vi "Add Cashier.vi"(7 "Time Scale [ms]":u32=3000, 8 "error in (no error)":errorcluster, 10 "Name":string, 11 "Coffee Shop in":refnum<class "Coffee Shop.lvclass">) -> (0 "error out":errorcluster, 3 "Coffee Shop out":refnum<class "Coffee Shop.lvclass">)   [LabVIEW 2020, in "Coffee Shop.lvclass"]
uses:
  Coffee Shop.lvclass
  C:/Program Files (x86)/National Instruments/LabVIEW 2020/vi.lib/Astemes/Triarc Framework/Process/Process.lvclass
  People/Workers/Cashier/Cashier.lvclass
  C:/git/astemes-triarc-examples/source/Coffee Shop/Processes/People/Person/Person.lvclass
  People/Person/Person.lvclass/Person.ctl
  <vilib>/Astemes/Triarc Framework/Process/Process.lvclass/Process.ctl
  <vilib>/Astemes/Triarc Framework/Process/Private/SubVIs/Handle Debug Data.vi
  <vilib>/Astemes/Triarc Framework/Logging/Log Debug.vi
  <vilib>/AdvancedString/1D String Array to Delimited String.vi
  <vilib>/Utility/High Resolution Relative Seconds.vi
  <vilib>/Astemes/Triarc Framework/Process/Public/Read Name.vi
  <vilib>/Astemes/Triarc Framework/Callback/Callback.lvclass
  Coffee Shop.lvclass/Coffee Shop.ctl
  <vilib>/Astemes/Triarc Framework/Process/Process.lvclass
  C:/git/astemes-triarc-examples/source/Coffee Shop/Processes/People/Workers/Worker/Worker.lvclass
  C:/Program Files (x86)/National Instruments/LabVIEW 2020/vi.lib/Astemes/Triarc Framework/View/View.lvclass
  C:/Program Files (x86)/National Instruments/LabVIEW 2020/vi.lib/Astemes/Triarc Framework/Base/Base.lvclass
  C:/Program Files (x86)/National Instruments/LabVIEW 2020/vi.lib/Astemes/Triarc Framework/Error Handler Interface/Error Handler Interface.lvclass
  C:/Program Files (x86)/National Instruments/LabVIEW 2020/vi.lib/Astemes/Triarc Framework/Logging/Logging.lvclass
  C:/git/astemes-triarc-examples/source/Coffee Shop/Processes/People/Process Job/Job Handler.lvclass
  C:/git/astemes-triarc-examples/source/Coffee Shop/Processes/People/Workers/Cashier/Cashier.lvclass
  People/Person/Person.lvclass
  C:/Program Files (x86)/National Instruments/LabVIEW 2020/vi.lib/Astemes/Triarc Framework/Application/Application.lvclass
  C:/Program Files (x86)/National Instruments/LabVIEW 2020/vi.lib/Astemes/Triarc Framework/Async Handler/Async Handler.lvclass
  C:/git/astemes-triarc-examples/source/Coffee Shop/Processes/Coffee Shop/Coffee Shop.lvclass
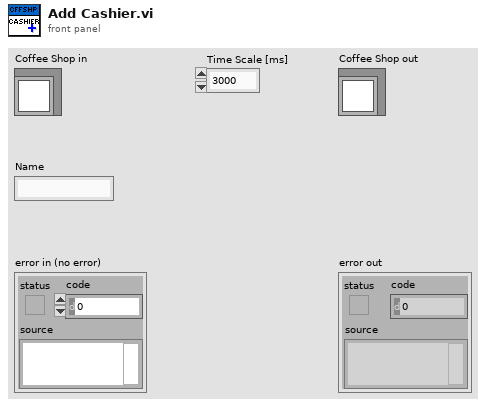
[diagram p1: front panel]
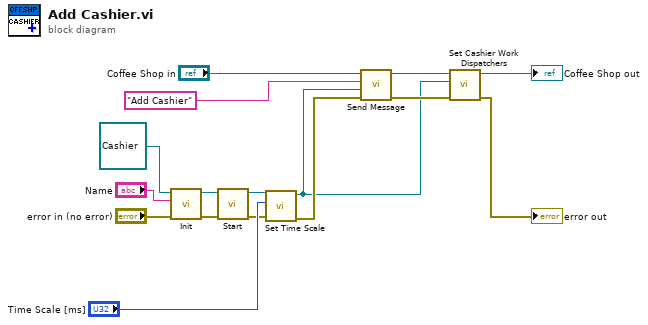
[diagram p0: block diagram]
diagram:
  n1 = call-dynamic "Init.vi"("error in (no error)"="error in (no error)", "Name"="Name", "View In"=refnum<class "Cashier.lvclass"> refnum ("Cashier.lvclass")) -> ("error out"=w10:errorcluster, "View Out"=w2:refnum<class "Cashier.lvclass">)  [unwired: 7 in]
  n2 = call <vilib>:"Start.vi"("error in (no error)"=w10, "Process In"=w2) -> ("error out"=w3:errorcluster, "Process Out"=w1:refnum<class "Cashier.lvclass">)  [unwired: 7 in, 1 out]
  n3 = call "Set Time Scale.vi"("TRIARC_ERROR_IN"=w3, "Time Scale [ms]"="Time Scale [ms]", "Person In"=w1) -> ("TRIARC_ERROR_OUT"=w6:errorcluster, "Person Out"=w5:refnum<class "Cashier.lvclass">)  [unwired: 7 in]
  n4 = call <vilib>:"Send Message.vi"("error in (no error)"=w6, "Message Data"=w5, "Message"="Add Cashier", "Process In"="Coffee Shop in") -> ("error out"=w16:errorcluster, "Process Out"=w8:refnum<class "Coffee Shop.lvclass">)  [unwired: 6 in]
  n5 = call "Set Cashier Work Dispatchers.vi"("error in (no error)"=w16, "Cashier"=w5, "Coffee Shop In"=w8) -> ("error out"=→"error out":errorcluster, "Coffee Shop Out"=→"Coffee Shop out":refnum<class "Coffee Shop.lvclass">)  [unwired: 7 in]
